vi "TrackingAppend.vi"(7 "Broadcast Length":i32, 9 "Timestamp":timestamp, 10 "Positions":dbl[][](array[numeric]), 11 "Position History":dbl[][](array[numeric])) -> (3 "Position History Out":dbl[][](array[numeric]))   [LabVIEW 2017, in "ImageAcquisitionLibrary.lvlib"]
uses:
  ImageAcquisitionProgram/ImageAcquisitionLibrary/ImageAcquisitionLibrary.lvlib
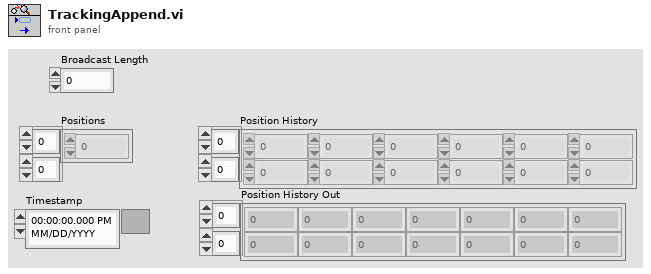
[diagram p1: front panel]
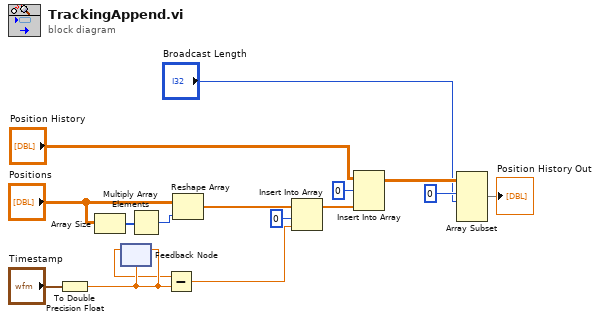
[diagram p0: block diagram]
diagram:
  n1 = To Double Precision Float(number="Timestamp") -> (double precision float=w10:dbl)
  n2 = Array Size(array="Positions") -> (size(s)=w15:i32[])
  n3 = feedback-in #1(w10) -> ()
  n4 = feedback #1(w10) -> (w9:dbl)
  n5 = Multiply Array Elements(1:w15) -> (0:w14:i32)
  n6 = Subtract(x=w9, y=w10) -> (x-y=w8:dbl)
  n7 = Reshape Array("Positions", w14) -> (w13:dbl[])
  n8 = Insert Into Array(array=w13, index=0, new element=w8) -> (w6:dbl[])
  n9 = Insert Into Array(array="Position History", index (row)=0, new element=w6) -> (w4:dbl[][])  [unwired: 1 in]
  n10 = Array Subset(array=w4, index (row)=0 ("index"), length (row)="Broadcast Length") -> (→"Position History Out":dbl[][])  [unwired: 2 in]
